vi "ADStar Navigation - Unknown Map.vi"() -> ()   [LabVIEW 2013]
doc: "This example continually replans a path from Start to Goal while following the best known path, including through obstacles if necessary.\nThe Anytime D* search algorithm is useful when the world or the robot's understanding of the world is changing. Anytime D* maintains more information than the A* search algorithm so the robot can backtrack and find a new path more easily if it discovers the original path will not work."
uses:
  <vilib>/robotics/Navigation/shared/WorldMap/OccupancyGridWorldMap/NI_Robotics_OccupancyGridWorldMap.lvclass
  <vilib>/robotics/Navigation/Anytime D Star/NI_Robotics_AnytimeDStar.lvclass
panel:
  in  "Random Obstacles?":bool
  in  "Step Through":bool
  in  "Sensor Radius":i32=5 min=0
  in  "% Random Obstacles":dbl=40.0 min=0.0 max=100.0 step=1.0 format="%#_3g"
  in  "goal y":i32=35
  in  "goal x":i32=50
  out "Open List Size":i32(graph)=1665
  out "path on obstacles":dbl[][](graph)
  out "AD* Open Nodes":i32=1665 caption="size"
  out "Path Cost":dbl(graph)
  in  "Epsilon":i32=2 min=1
  out "AD* Path Cost":dbl caption="path cost"
  in  "y start":i32
  in  "x start":i32
  in  "Move Robot":i32=1 min=0
  in  "Overhaul":i32=25
  in  "step button":bool
  out "AD* Time":u32=117 caption="seconds"
  out "Compute Path Time":u32(graph)=117
  in  "stop":bool
  # "The Anytime D* search algorithm is useful when the world or the robot's understanding of the world is changing.  Anytime D* maintains more information\n than the A* search algorithm so the robot can backtrack and find a new path more easily if it discovers the original path will not work."
  # "This example continually replans a path from Start to Goal while \nfollowing the best known path, including through obstacles if necessary."
  # "Configuration"
  # "X"
  # "Y"
  # "Start"
  # "Goal"
  # "Run Mode"
  # "Run-time Control"
  # "Detection radius of robot's sensors."
  # "Number of steps the robot takes after each plan."
  # "Number of steps before AD* plans from scratch."
  # "1) Choose the Start and Goal location and the % Random Obstacles.\n2) Run the VI.\n3) Adjust the controls in the Run-time Controls section to see the \n     effect each option has on path planning\n4) Change the Run Mode to Single Step to pause after each time\n the AD* VI runs"
  # "A higher epsilon results in a faster but less optimal search."
  # "Continuous"
  # "Single Step"
  # "Robot"
  # "Obstacle"
  # "Unknown"
  # "Free"
  # "Path"
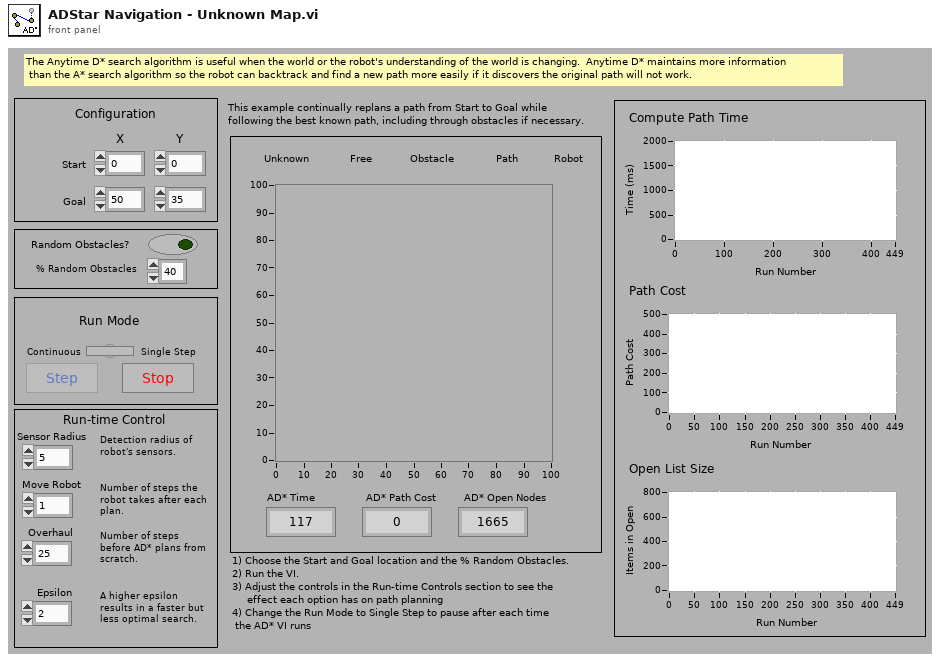
[diagram p1: front panel]
types:
  T1 = enum8{"Enabled", "Disabled", "Disabled and Grayed Out"}
  T2 = cluster{"epsilon":dbl, "run number":i32, "open list size":i32}
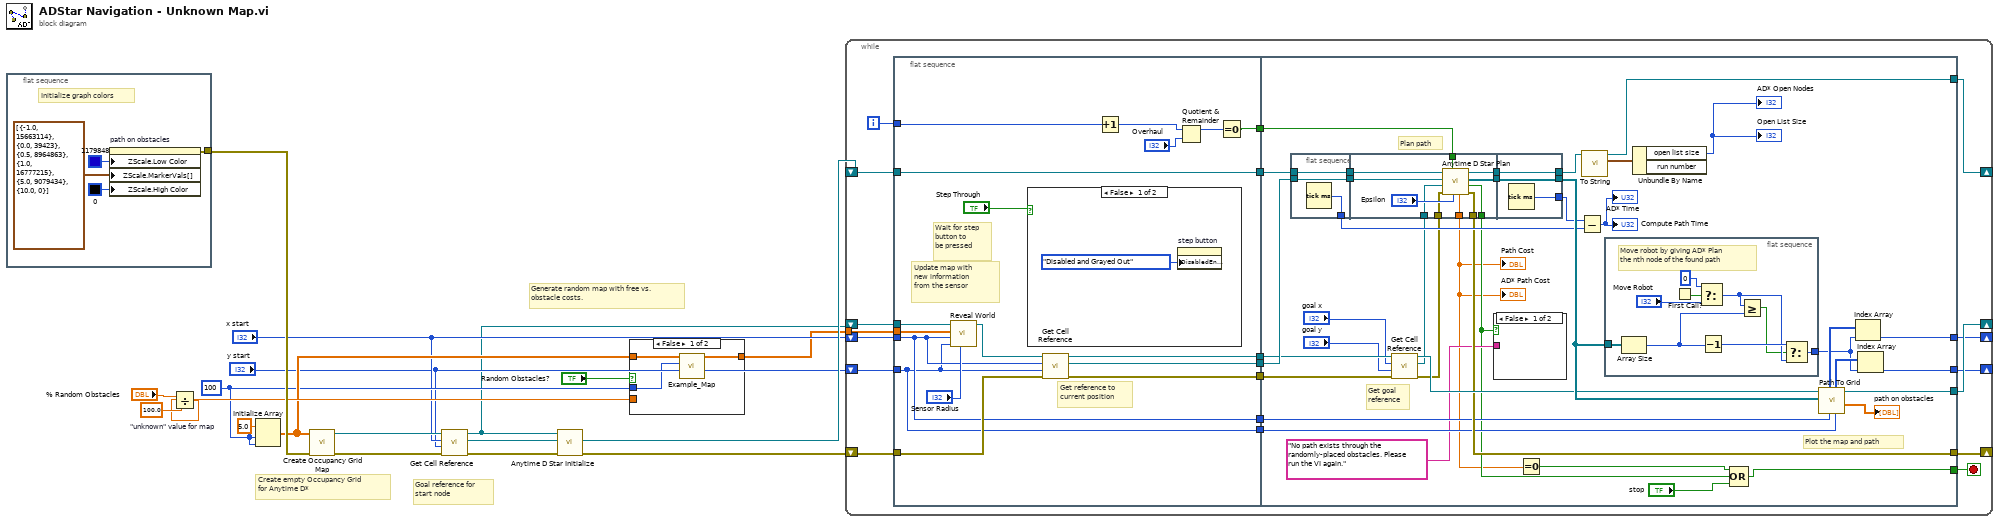
[diagram p0: block diagram]
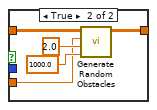
[diagram p2: hidden frame]
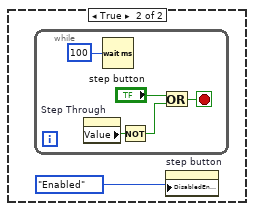
[diagram p3: hidden frame]
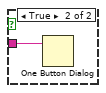
[diagram p4: hidden frame]
diagram:
  w6 = 100 ("dimension size")
  w17 = 5.0  # "unknown" value for map
  # "Goal reference for\nstart node"
  # "Generate random map with free vs.\nobstacle costs."
  # "Create empty Occupancy Grid\nfor Anytime D*"
  n1 = flat-sequence {
    tunnel: [w19] -> w11
    frame #0 {
      # "Initialize graph colors"
      n2 = property on="path on obstacles" class="IntGraph (strict)"("ZScale.Low Color"=u32 1179848, "ZScale.MarkerVals[]"=cluster{dbl, u32}[] [{-1.0, 15663114}, {0.0, 39423}, {0.5, 8964863}, {1.0, 16777215}, {5.0, 9079434}, {10.0, 0}], "ZScale.High Color"=u32 0) -> (error out=w19:errorcluster)  [unwired: 2 in, 1 out]
    }
  }
  n3 = Divide(x="% Random Obstacles", y=100.0) -> (x/y=w8:dbl)
  n4 = Initialize Array(w17, w6, w6) -> (w7:dbl[][])
  n5 = call <vilib>:"Create Occupancy Grid Map.vi"("error in (no error)"=w11, "occupancy grid"=w7) -> ("error out"=w14:errorcluster, "map reference out"=w15:refnum<data-value>)  [unwired: 8 in]
  n6 = call <vilib>:"Get Cell Reference.vi"("error in (no error)"=w14, "y"="y start", "x"="x start", "map reference in"=w15) -> ("error out"=w13:errorcluster, "cell reference"=w16:refnum<data-value>, "map reference out"=w2:refnum<data-value>)  [unwired: 4 in, 1 out]
  n7 = call <vilib>:"Anytime D Star Initialize.vi"("error in (no error)"=w13, "start reference"=w16, "map reference in"=w2) -> ("error out"=w12:errorcluster, "Anytime D*"=w10:refnum<class "NI_Robotics_AnytimeDStar.lvclass">)  [unwired: 7 in]
  n8 = case shown="False" "Random Obstacles?" {
    tunnel: w8 -> [_ w28]
    tunnel: w7 -> [w25 w27]
    tunnel: [w24 w26] -> w1
    tunnel: w6 -> [w23 _]
    frame False {
      n9 = call "Example_Map.vi"("dimension size"=w23, "Array in"=w25) -> ("Array out"=w24:dbl[][])  [unwired: 9 in]
    }
    frame True {
      n10 = call "Generate Random Obstacles.vi"("obstacle cost"=1000.0, "free cost"=2.0, "chance"=w28, "cost in"=w27) -> ("cost out"=w26:dbl[][])  [unwired: 7 in]
    }
  }
  n11 = while {
    shift-right: [w40] -> _
    shift-left: w10 -> [w50]
    shift-right: [w48] -> _
    shift-left: w2 -> [w49]
    tunnel: w1 -> [w43]
    shift-right: [w39] -> _
    shift-left: "x start" -> [w42]
    shift-right: [w38] -> _
    shift-left: "y start" -> [w41]
    shift-right: [w33] -> _
    shift-left: w12 -> [w35]
    i -> [w37]
    stop <- w47 stop-if-true
    n12 = flat-sequence {
      tunnel: w37 -> [w56]
      tunnel: w49 -> [w64]
      tunnel: w50 -> [w67]
      tunnel: [w67] -> w46
      tunnel: [w62] -> w45
      tunnel: [w61] -> w44
      tunnel: w43 -> [w66]
      tunnel: w42 -> [w52]
      tunnel: w41 -> [w51]
      tunnel: [w55] -> w36
      tunnel: w35 -> [w54]
      tunnel: [w53] -> w34
      tunnel: [w52] -> w32
      tunnel: [w51] -> w31
      tunnel: [w77] -> w47
      tunnel: [w111] -> w40
      tunnel: [w99] -> w48
      tunnel: [w92] -> w39
      tunnel: [w91] -> w38
      tunnel: w36 -> [w97]
      tunnel: w44 -> [w96]
      tunnel: w45 -> [w90]
      tunnel: w46 -> [w107]
      tunnel: w34 -> [w87]
      tunnel: [w83] -> w33
      tunnel: w32 -> [w82]
      tunnel: w31 -> [w81]
      frame #0 {
        # "Get reference to \ncurrent position"
        # "Update map with new information\nfrom the sensor"
        # "Wait for step\nbutton to\nbe pressed"
        n13 = call "Reveal World.vi"("radius"="Sensor Radius", "y"=w51, "x"=w52, "cost in"=w66, "map reference in"=w64) -> ("map reference in 2"=w63:refnum<data-value>)  [unwired: 5 in, 1 out]
        n14 = case shown="False" "Step Through" {
          frame False {
            n15 = property on="step button" class="Bool (strict)"("DisabledEnum"=T1."Disabled and Grayed Out" ("Disabled")) -> ()  [unwired: 2 in, 2 out]
          }
          frame True {
            n16 = while {
              stop <- w72 stop-if-true
              n17 = property on="Step Through" class="Bool (strict)"() -> ("Value"=w70:bool)  [unwired: 2 in, 2 out]
              n18 = Wait (ms)(milliseconds to wait=u32 100) -> ()  [unwired: 1 out]
              n19 = Not(x=w70) -> (.not. x?=w71:bool)
              n20 = Or(x="step button", y=w71) -> (x .or. y?=w72:bool)
            }
            n21 = property on="step button" class="Bool (strict)"("DisabledEnum"=T1."Enabled" ("Disabled")) -> ()  [unwired: 2 in, 2 out]
          }
        }
        n22 = call <vilib>:"Get Cell Reference.vi"("error in (no error)"=w54, "y"=w51, "x"=w52, "map reference in"=w63) -> ("error out"=w53:errorcluster, "cell reference"=w61:refnum<data-value>, "map reference out"=w62:refnum<data-value>)  [unwired: 4 in, 1 out]
        n23 = Increment(x=w56) -> (x+1=w58:i32)
        n24 = Quotient & Remainder(x=w58, y="Overhaul") -> (x-y*floor(x/y)=w57:i32)  [unwired: 1 out]
        n25 = Equal To 0?(x=w57) -> (x = 0?=w55:bool)
      }
      frame #1 {
        # "Plot the map and path"
        # "Get goal \nreference"
        # "Plan path"
        n26 = flat-sequence {
          tunnel: w107 -> [w124]
          tunnel: w96 -> [w125]
          tunnel: [w125] -> w106
          tunnel: [w124] -> w105
          tunnel: [w123] -> w101
          tunnel: [w132] -> w78
          tunnel: [w131] -> w76
          tunnel: w106 -> [w135]
          tunnel: w105 -> [w136]
          tunnel: [w133] -> w104
          tunnel: [w134] -> w103
          tunnel: w97 -> [w129]
          tunnel: w85 -> [w128]
          tunnel: w84 -> [w127]
          tunnel: [w126] -> w83
          tunnel: [w138] -> w110
          tunnel: [w139] -> w112
          tunnel: w104 -> [w139]
          tunnel: w103 -> [w138]
          tunnel: [w137] -> w102
          frame #0 {
            n27 = Tick Count (ms)() -> (millisecond timer value=w123:u32)
          }
          frame #1 {
            n28 = call <vilib>:"Anytime D Star Plan.vi"("epsilon"="Epsilon", "overhaul (F)"=w129, "error in (no error)"=w127, "new goal reference"=w128, "current reference"=w135, "Anytime D* in"=w136) -> ("error out"=w126:errorcluster, "no valid path exists"=w132:bool, "path references"=w134:refnum<data-value>[], "Anytime D* out"=w133:refnum<class "NI_Robotics_AnytimeDStar.lvclass">, "path cost"=w131:dbl)  [unwired: 1 in]
          }
          frame #2 {
            n29 = Tick Count (ms)() -> (millisecond timer value=w137:u32)
          }
        }
        n30 = call <vilib>:"Get Cell Reference.vi"("error in (no error)"=w87, "y"="goal y", "x"="goal x", "map reference in"=w90) -> ("error out"=w84:errorcluster, "cell reference"=w85:refnum<data-value>, "map reference out"=w86:refnum<data-value>)  [unwired: 4 in, 1 out]
        n31 = case shown="False" w78 {
          tunnel: "No path exists through the randomly-placed obstacles. Please run the VI again." -> [_ w113]
          frame False {
          }
          frame True {
            n32 = One Button Dialog(message=w113) -> ()  [unwired: 1 in, 1 out]
          }
        }
        n33 = Equal To 0?(x=w76) -> (x = 0?=w75:bool)
        n34 = Subtract(x=w102, y=w101) -> (x-y=→"Compute Path Time" →"AD* Time":u32)
        n35 = call <vilib>:"To String.vi"("Anytime D* in"=w112) -> ("output"=w109:T2, "Anytime D* out"=w111:refnum<class "NI_Robotics_AnytimeDStar.lvclass">)  [unwired: 8 in, 1 out]
        n36 = flat-sequence {
          tunnel: w110 -> [w121]
          tunnel: [w114] -> w93
          frame #0 {
            # "Move robot by giving AD* Plan\nthe nth node of the found path"
            n37 = Array Size(array=w121) -> (size(s)=w118:i32)
            n38 = First Call?() -> (First Call?: T/F=w120:bool)
            n39 = Select(t=0, s=w120, f="Move Robot") -> (s? t:f=w117:i32)
            n40 = Decrement(x=w118) -> (x-1=w122:i32)
            n41 = Greater Or Equal?(x=w117, y=w118) -> (x >= y?=w116:bool)
            n42 = Select(t=w122, s=w116, f=w117) -> (s? t:f=w114:i32)
          }
        }
        n43 = Unbundle By Name(w109) -> ("open list size"=→"Open List Size" →"AD* Open Nodes":i32)  [unwired: 1 out]
        n44 = Compound Arithmetic op=OR(w75, w78, "stop") -> (w77:bool)
        n45 = call "Path To Grid.vi"("current y"=w81, "current x"=w82, "path references"=w110, "map reference in"=w86) -> ("path on obstacles"=→"path on obstacles":dbl[][], "map reference out"=w99:refnum<data-value>, "y coordinates"=w95:i32[], "x coordinates"=w94:i32[])  [unwired: 3 in, 1 out]
        n46 = Index Array(array=w94, index=w93) -> (element=w92:i32)
        n47 = Index Array(array=w95, index=w93) -> (element=w91:i32)
        "AD* Path Cost" <- w76
        "Path Cost" <- w76
      }
    }
  }
